vi "TaggerRbRy.vi"() -> ()   [LabVIEW 2013]
uses:
  Shared Libraries/Controls/FileName_Cluster.ctl
  <vilib>/addons/h5labview2/file/H5Fmode.ctl
  <vilib>/addons/h5labview2/base/lib_path.vi
  <vilib>/addons/h5labview2/base/H5Equery.vi
  <vilib>/addons/h5labview2/base/hid_t.ctl
  <vilib>/addons/h5labview2/dataset/H5Dwrite.llb/H5Dwrite.xnode
  <vilib>/addons/h5labview2/file/H5F.lvlib
  <vilib>/addons/h5labview2/group/H5G.lvlib
panel:
  out "concatenated string":string
  in  "Stop":bool
  in  "?":enum32{"Control", "Error"}(tab)
  in  "Trigger Level (mV)":u16=500
  in  "Processing Delay":u32=250
  in  "ClockLine":u16=2
  in  "Channel List":u8[](array[numeric])
  in  "Analysis type":T1(ring)
  in  "Measurement Windows":u16=3
  in  "# of shots to average over":u16=1
  out "Tagger loop":u32
  in  "Tagger IP address":string="192.168.1.115"
  in  "Get Setlist inform string":bool=TRUE
  out "Inform string":string
  in  "Do Matlab Analysis":bool
  out "Matlab Command":string
  in  "Save Experimental Parameters to file":enum16{"False", "True"}(ring)
  in  "Save permanent file?":bool=TRUE
  in  "File Paramaters":T2={"Data Root"=path "C:/Data", "Index"=0, "Instrument"="TTM8000"} {"Index" format="%04d"}
  out "exe error":errorcluster
  out "HDF5 error":errorcluster
  out "command output":string
  out "move error out":errorcluster
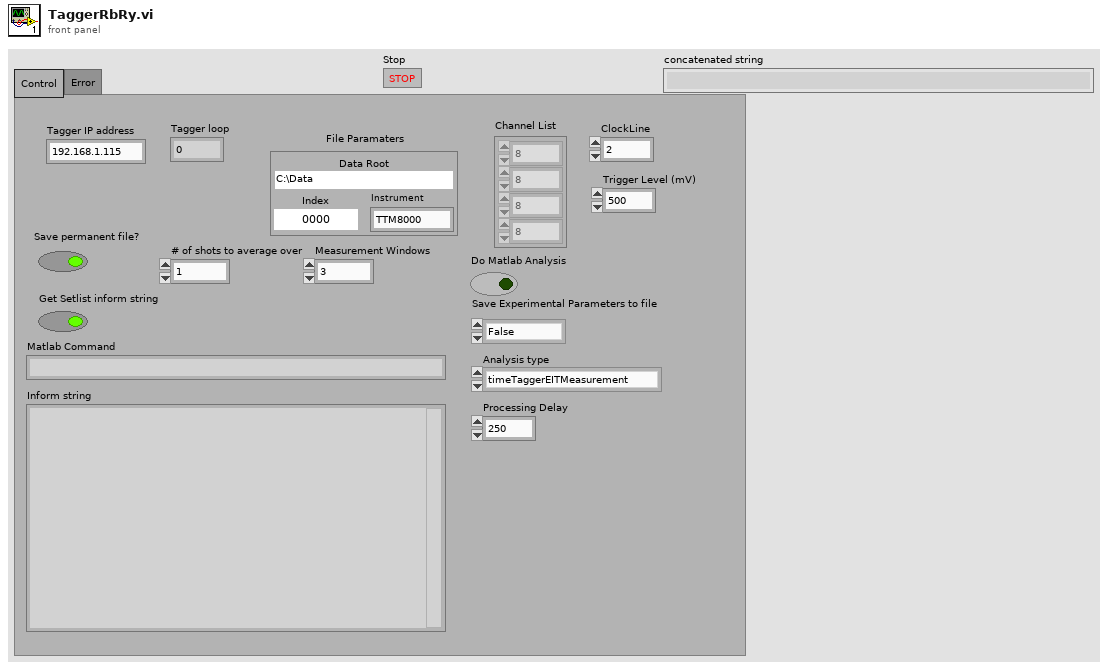
[diagram p1: front panel]
types:
  T1 = enum16{"timeTaggerEITMeasurement", "timeTaggerODMeasurement", "timeTaggerDoubleODMeasurement", "timeTaggerSpectra", "runningG2", "timeTaggerPulseMeasurement"}
  T2 = typedef "FileName_Cluster.ctl" = cluster{"Data Root":path, "Index":u32, "Instrument":string}
  T3 = enum16{"open", "replace", "create", "open or create", "replace or create", "replace or create with confirmation"}
  T4 = typedef "H5F.lvlib/H5Fmode.ctl" = enum16{"read-only", "read-write", "overwrite", "create new", "open or create"}
  T5 = typedef "hid_t.ctl" = i32
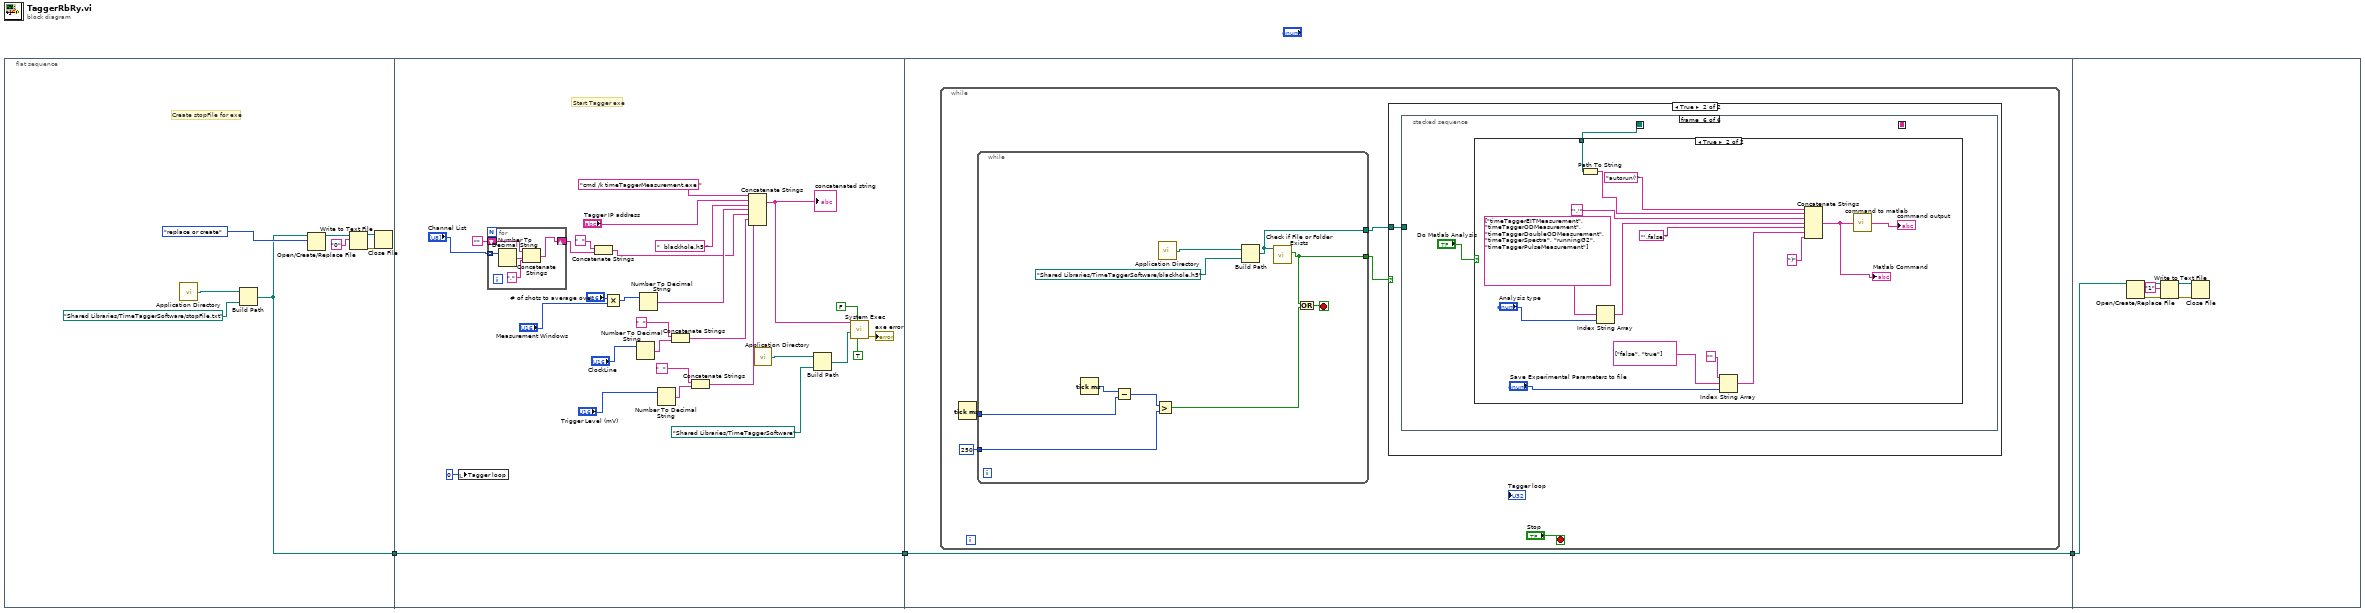
[diagram p0: block diagram]
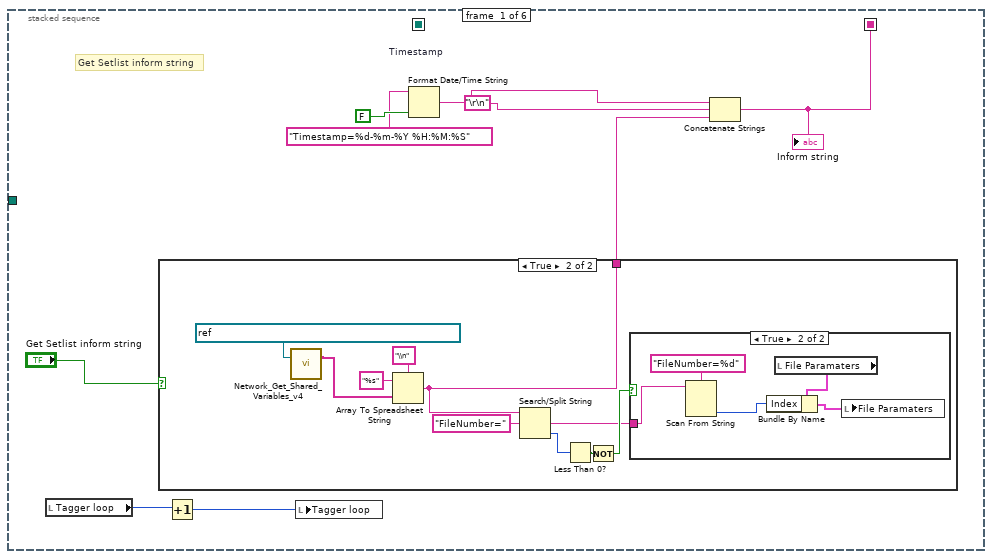
[diagram p3: hidden frame]
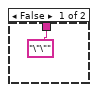
[diagram p4: hidden frame]
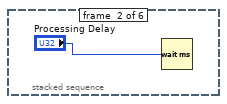
[diagram p6: hidden frame]
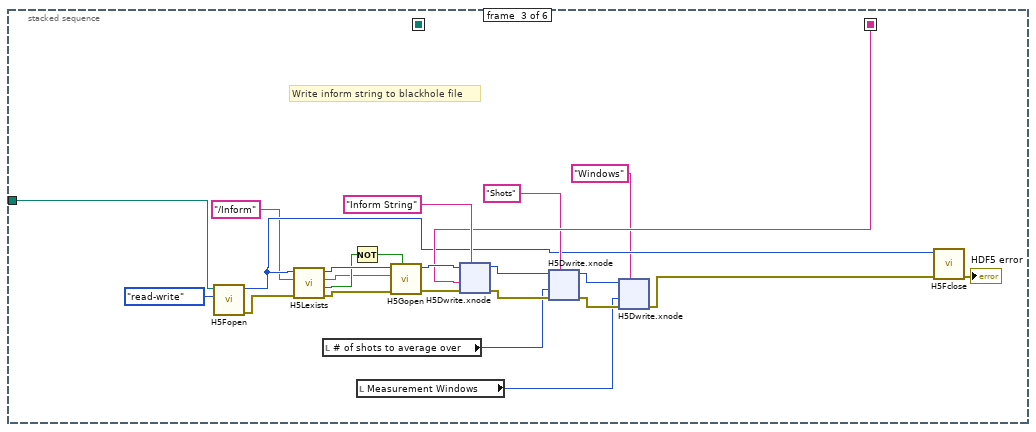
[diagram p7: hidden frame]
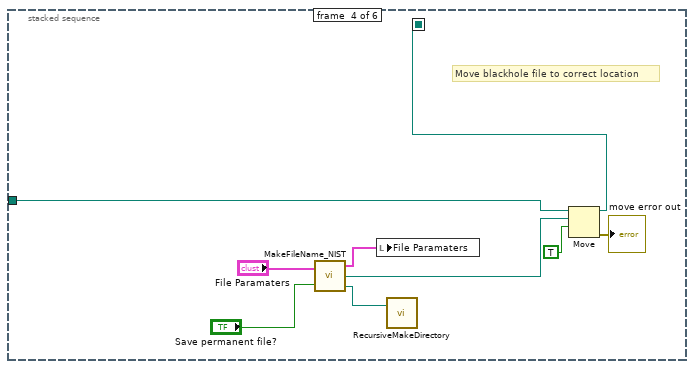
[diagram p8: hidden frame]
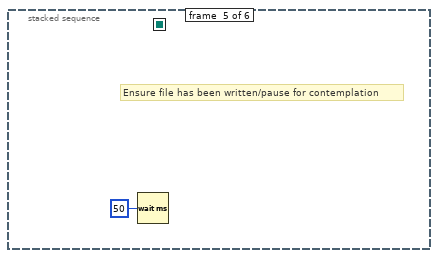
[diagram p9: hidden frame]
diagram:
  n1 = flat-sequence {
    tunnel: [w4] -> w1
    tunnel: [w29] -> w2
    tunnel: w1 -> [w29]
    tunnel: [w46] -> w3
    tunnel: w2 -> [w46]
    tunnel: w3 -> [w199]
    frame #0 {
      # "Create stopFile for exe"
      n2 = call <vilib>:"Application Directory.vi"() -> ("Application Directory"=w10:path)
      n3 = Build Path(base path=w10, name or relative path=path "Shared Libraries/TimeTaggerSoftware/stopFile.txt" ("working directory")) -> (appended path=w4:path)
      n4 = Open/Create/Replace File(file path (use dialog)=w4, operation (0:open)=T3."replace or create") -> (refnum out=w9:refnum<file>)  [unwired: 4 in, 2 out]
      n5 = Write to Text File(file (use dialog)=w9, text="0") -> (refnum out=w6:refnum<file>, error out=w5:errorcluster)  [unwired: 2 in, 1 out]
      n6 = Close File(refnum=w6, error in=w5) -> ()  [unwired: 2 out]
    }
    frame #1 {
      # "Start Tagger exe"
      n7 = local write "Tagger loop"(u32 0 ("Tagger loop")) -> ()
      n8 = for {
        tunnel: "Channel List" -> [w43] mode=indexing
        shift-right: [w44] -> w23
        shift-left: "" -> [w45]
        n9 = Number To Decimal String(number=w43) -> (decimal integer string=w42:string)  [unwired: 1 in]
        n10 = Concatenate Strings(w45, w42, "," ("string")) -> (w44:string)
      }
      n11 = Concatenate Strings("  " ("string"), w23) -> (w21:string)
      n12 = Multiply(x="# of shots to average over", y="Measurement Windows") -> (x*y=w26:u16)
      n13 = Number To Decimal String(number="ClockLine") -> (decimal integer string=w18:string)  [unwired: 1 in]
      n14 = Number To Decimal String(number=w26) -> (decimal integer string=w28:string)  [unwired: 1 in]
      n15 = Number To Decimal String(number="Trigger Level (mV)") -> (decimal integer string=w15:string)  [unwired: 1 in]
      n16 = Concatenate Strings("  " ("string"), w18) -> (w16:string)
      n17 = Concatenate Strings("  " ("string"), w15) -> (w12:string)
      n18 = Concatenate Strings("cmd /k timeTaggerMeasurement.exe " ("string"), "Tagger IP address", "  blackhole.h5 " ("string"), w28, w21, w16, w12) -> (w31:string)
      "concatenated string" <- w31
      n19 = call <vilib>:"Application Directory.vi"() -> ("Application Directory"=w38:path)
      n20 = Build Path(base path=w38, name or relative path=path "Shared Libraries/TimeTaggerSoftware" ("working directory")) -> (appended path=w40:path)
      n21 = call <vilib>:"System Exec.vi"("run minimized? (F)"=TRUE, "wait until completion? (T)"=FALSE, "working directory"=w40, "command line"=w31) -> ("error out"=→"exe error":errorcluster)  [unwired: 4 in, 3 out]
    }
    frame #2 {
      n22 = while {
        stop <- "Stop" stop-if-true
        n23 = Tick Count (ms)() -> (millisecond timer value=w48:u32)
        n24 = while {
          tunnel: [w191] -> w49
          tunnel: [w185] -> w50
          tunnel: w48 -> [w189]
          tunnel: u32 250 -> [w187]
          stop <- w186 stop-if-true
          n25 = Tick Count (ms)() -> (millisecond timer value=w190:u32)
          n26 = Subtract(x=w190, y=w189) -> (x-y=w188:u32)
          n27 = Greater?(x=w188, y=w187) -> (0:w184:bool)
          n28 = call <vilib>:"Application Directory.vi"() -> ("Application Directory"=w193:path)
          n29 = Build Path(base path=w193, name or relative path=path "Shared Libraries/TimeTaggerSoftware/blackhole.h5" ("working directory")) -> (appended path=w191:path)
          n30 = call <vilib>:"Check if File or Folder Exists.vi"("path"=w191) -> ("file or folder exists?"=w185:bool)  [unwired: 8 in, 2 out]
          n31 = Or(x=w185, y=w184) -> (x .or. y?=w186:bool)
        }
        n32 = case shown="True" w50 {
          tunnel: w49 -> [_ w52]
          frame False {
          }
          frame True {
            n33 = stacked-sequence {
              seq-local: [w53 _ _ _ _ _] -> [_ _ w98 _ _ _]
              seq-local: [_ _ _ w159 _ _] -> [_ _ _ _ _ w167]
              tunnel: w52 -> [_ _ w96 w162 _ _]
              frame #0 {
                # "Get Setlist inform string"
                n34 = local read "Tagger loop"() -> (w60:u32)
                n35 = case shown="True" "Get Setlist inform string" {
                  tunnel: ["\"\"" ("spreadsheet string") w63] -> w55
                  frame False {
                  }
                  frame True {
                    n36 = call "Network_Get_Shared_Variables_v4.vi"("Source of Data"=refnum<k21> "\\\\localhost\\VariableLibrary\\Instruction String") -> ("Igor Instruction String"=w65:string[])  [unwired: 1 in, 1 out]
                    n37 = Array To Spreadsheet String(delimiter (Tab)="\\n", array=w65, 3:"%s" ("format string")) -> (spreadsheet string=w63:string)
                    n38 = Search/Split String(string=w63, search string/char (-)="FileNumber=") -> (match + rest of string=w64:string, offset of match=w69:i32)  [unwired: 1 in, 1 out]
                    n39 = Less Than 0?(x=w69) -> (x < 0?=w68:bool)
                    n40 = Not(x=w68) -> (.not. x?=w67:bool)
                    n41 = case shown="True" w67 {
                      tunnel: w64 -> [_ w76]
                      frame False {
                      }
                      frame True {
                        n42 = Scan From String(format string="FileNumber=%d", input string=w76) -> (output 1=w75:i32)  [unwired: 2 in, 4 out]
                        n43 = local read "File Paramaters"() -> (w73:T2)
                        n44 = Bundle By Name(cluster=w73, "Index"=w75) -> (w74:T2)
                        n45 = local write "File Paramaters"(w74) -> ()
                      }
                    }
                  }
                }
                n46 = Increment(x=w60) -> (x+1=w59:u32)
                n47 = local write "Tagger loop"(w59) -> ()
                n48 = Format Date/Time String "Timestamp"(time format string (%c)="Timestamp=%d-%m-%Y %H:%M:%S", UTC format=FALSE) -> (date/time string=w56:string)  [unwired: 1 in]
                n49 = Concatenate Strings(w56, "\r\n", w55) -> (w53:string)
                "Inform string" <- w53
              }
              frame #1 {
                n50 = Wait (ms)(milliseconds to wait="Processing Delay") -> ()  [unwired: 1 out]
              }
              frame #2 {
                # "Write inform string to blackhole file"
                n51 = call <vilib>:"H5Fopen.vi"("mode (read-only)"=H5Fmode."read-write", "path"=w96) -> ("error out"=w88:errorcluster, "ref out"=w91:T5)  [unwired: 8 in]
                n52 = call <vilib>:"H5Lexists.vi"("error in (no error)"=w88, "path"="/Inform" ("name"), "ref in"=w91) -> ("error out"=w89:errorcluster, "exists?"=w86:bool, "path out"=w80:string, "ref out"=w90:T5)  [unwired: 5 in]
                n53 = local read "# of shots to average over"() -> (w93:u16)
                n54 = Not(x=w86) -> (.not. x?=w85:bool)
                n55 = local read "Measurement Windows"() -> (w81:u16)
                n56 = call <vilib>:"H5Gopen.vi"("create? (F)"=w85, "error in (no error)"=w89, "name"=w80, "ref in"=w90) -> ("error out"=w99:errorcluster, "group out"=w101:T5)  [unwired: 6 in]
                n57 = xnode "H5Dwrite.xnode"("dataset name"="Inform String", "error in (no error)"=w99, "data"=w98, "ref in"=w101) -> ("error out"=w94:errorcluster, "ref out"=w95:T5)  [unwired: 3 in, 1 out]
                n58 = xnode "H5Dwrite.xnode"("dataset name"="Shots", "error in (no error)"=w94, "data"=w93, "ref in"=w95) -> ("error out"=w83:errorcluster, "ref out"=w84:T5)  [unwired: 3 in, 1 out]
                n59 = xnode "H5Dwrite.xnode"("dataset name"="Windows", "error in (no error)"=w83, "data"=w81, "ref in"=w84) -> ("error out"=w79:errorcluster)  [unwired: 3 in, 2 out]
                n60 = call <vilib>:"H5Fclose.vi"("error in (no error)"=w79, "ref"=w91) -> ("error out"=→"HDF5 error":errorcluster)  [unwired: 9 in]
              }
              frame #3 {
                # "Move blackhole file to correct location"
                n61 = call "MakeFileName_NIST.vi"("File Parameters"="File Paramaters", "Save permanent file?"="Save permanent file?") -> ("New file parameters."=w163:T2, "Path to File"=w161:path, "path"=w158:path)
                n62 = local write "File Paramaters"(w163) -> ()
                n63 = call "RecursiveMakeDirectory.vi"("Directory to create"=w158) -> ()  [unwired: 1 in, 2 out]
                n64 = Move(source path=w162, 9:TRUE ("overwrite (F)"), 10:w161) -> (error out=→"move error out":errorcluster, 3:w159:path)  [unwired: 2 in, 1 out]
              }
              frame #4 {
                # "Ensure file has been written/pause for contemplation"
                n65 = Wait (ms)(milliseconds to wait=u32 50) -> ()  [unwired: 1 out]
              }
              frame #5 {
                n66 = case shown="True" "Do Matlab Analysis" {
                  tunnel: w167 -> [_ w183]
                  frame False {
                  }
                  frame True {
                    n67 = Path To String(path=w183) -> (string=w181:string)
                    n68 = Index String Array(1:"Analysis type", 2:string[] ["timeTaggerEITMeasurement", "timeTaggerODMeasurement", "timeTaggerDoubleODMeasurement", "timeTaggerSpectra", "runningG2", "timeTaggerPulseMeasurement"] ("string array")) -> (0:w169:string)  [unwired: 1 in]
                    n69 = Index String Array(1:"Save Experimental Parameters to file", 2:string[] ["false", "true"] ("string array"), 3:"" ("string (\"\")")) -> (0:w175:string)
                    n70 = Concatenate Strings("autorun('" ("string"), w181, "','" ("string"), w169, "',false," ("string"), w175, ")" ("string")) -> (w173:string)
                    "Matlab Command" <- w173
                    n71 = call "command to matlab.vi"("matlabCommand"=w173) -> ("standard output"=→"command output":string)
                  }
                }
              }
            }
          }
        }
      }
    }
    frame #3 {
      n72 = Open/Create/Replace File(file path (use dialog)=w199) -> (refnum out=w197:refnum<file>, error out=w198:errorcluster)  [unwired: 5 in, 1 out]
      n73 = Write to Text File(file (use dialog)=w197, text="1", error in=w198) -> (refnum out=w194:refnum<file>, error out=w195:errorcluster)  [unwired: 1 in, 1 out]
      n74 = Close File(refnum=w194, error in=w195) -> ()  [unwired: 2 out]
    }
  }
